vi "DCA Close Test.vi"(6 "Driver Refs":T5, 8 "error in (no error)":errorcluster, 11 "Saved Instrument Configurations":cluster{"DMM Stimulus":T1, "SWI Position":T2}) -> (0 "error out":errorcluster {"code" format="%.0x"})   [LabVIEW 2011]
uses:
  drivers/DMM/DMM Driver Ref.ctl
  drivers/SWI/SWI Driver Ref.ctl
  TypeDefs/DCA Stimulus Parameters.ctl
  drivers/SWI/Sea-Level/TypeDefs/Sea-Level SWI Position.ctl
  drivers/DMM/DMM Command.ctl
  drivers/SWI/SWI Command.ctl
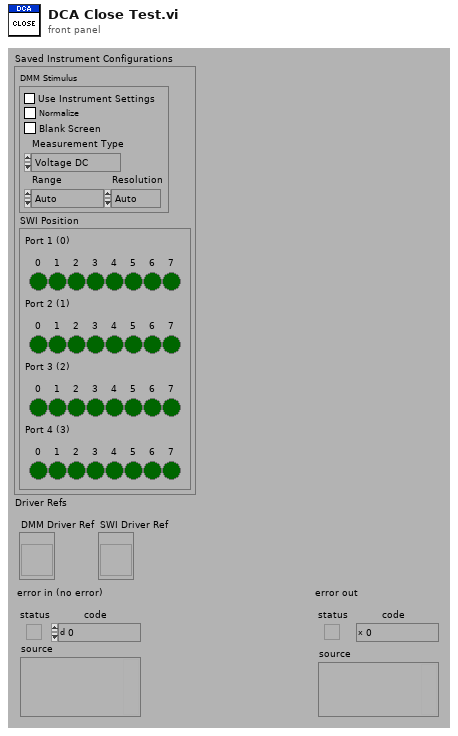
[diagram p1: front panel]
types:
  T1 = typedef "DCA Stimulus Parameters.ctl" = cluster{"Use Instrument":bool, "Normalize":bool, "Blank Screen":bool, "Measurement Type":enum16{"Voltage DC", "Voltage DC Ratio", "Voltage AC", "Current DC", "Current AC", "Resistance", "Fresistance", "Frequency", "Period", "Continuity", "Diode"}, "Range":enum16{"Auto", "Minimum", "Maximum", "100", "1,000", "10,000", "100,000", "1,000,000", "10,000,000", "100,000,000"}, "Resolution":enum16{"Auto", "4 1/2", "5 1/2", "6 1/2"}}
  T2 = typedef "Sea-Level SWI Position.ctl" = cluster{"Port 1 (0)":cluster{"0":bool, "1":bool, "2":bool, "3":bool, "4":bool, "5":bool, "6":bool, "7":bool}, "Port 2 (1)":cluster{"0":bool, "1":bool, "2":bool, "3":bool, "4":bool, "5":bool, "6":bool, "7":bool}, "Port 3 (2)":cluster{"0":bool, "1":bool, "2":bool, "3":bool, "4":bool, "5":bool, "6":bool, "7":bool}, "Port 4 (3)":cluster{"0":bool, "1":bool, "2":bool, "3":bool, "4":bool, "5":bool, "6":bool, "7":bool}}
  T3 = typedef "DMM Driver Ref.ctl" = refnum<vi>
  T4 = typedef "SWI Driver Ref.ctl" = refnum<vi>
  T5 = cluster{"DMM Driver Ref":T3, "SWI Driver Ref":T4}
  T6 = typedef "SWI Command.ctl" = enum16{"LOAD", "INITIALIZE", "PRESET", "SET STIMULUS", "GET STIMULUS", "GET INFO", "RELEASE", "UNLOAD"}
  T7 = typedef "DMM Command.ctl" = enum16{"LOAD", "INITIALIZE", "PRESET", "GET STIMULUS", "SET STIMULUS", "MEASURE", "RELEASE", "UNLOAD", "GET CALIBRATION", "CALIBRATE"}
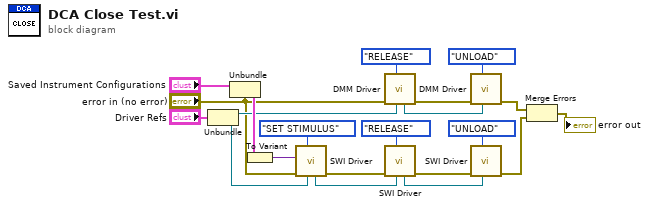
[diagram p0: block diagram]
diagram:
  n1 = Unbundle("Driver Refs") -> ("DMM Driver Ref"=w3:T3, "SWI Driver Ref"=w5:T4)
  n2 = Unbundle("Saved Instrument Configurations") -> ("SWI Position"=w6:T2)  [unwired: 1 out]
  n3 = To Variant(anything=w6) -> (Variant=w1:variant)
  n4 = call "SWI Driver.vi"("Drv Refnum"=w5, "SWI Command"=SWI_Command."SET STIMULUS", "error in (no error)"="error in (no error)", "SWI Position In"=w1) -> ("error out"=w8:errorcluster, "dup Drv Refnum"=w4:T4)  [unwired: 1 in, 5 out]
  n5 = call "DMM Driver.vi"("Drv Refnum"=w3, "DMM Command"=DMM_Command."RELEASE", "error in (no error)"="error in (no error)") -> ("error out"=w16:errorcluster, "dup Drv Refnum"=w14:T3)  [unwired: 2 in, 5 out]
  n6 = call "SWI Driver.vi"("Drv Refnum"=w4, "SWI Command"=SWI_Command."RELEASE", "error in (no error)"=w8) -> ("error out"=w17:errorcluster, "dup Drv Refnum"=w13:T4)  [unwired: 2 in, 5 out]
  n7 = call "DMM Driver.vi"("Drv Refnum"=w14, "DMM Command"=DMM_Command."UNLOAD", "error in (no error)"=w16) -> ("error out"=w12:errorcluster)  [unwired: 2 in, 6 out]
  n8 = call "SWI Driver.vi"("Drv Refnum"=w13, "SWI Command"=SWI_Command."UNLOAD", "error in (no error)"=w17) -> ("error out"=w11:errorcluster)  [unwired: 2 in, 6 out]
  n9 = Merge Errors(w12, w11) -> (→"error out":errorcluster)
